vi "set default configuration.vi"(8 "error in":errorcluster, 11 "Shared Memory configuration in":refnum<class "Shared Memory configuration.lvclass">) -> (0 "error out":errorcluster, 3 "Shared Memory configuration out":refnum<class "Shared Memory configuration.lvclass">)   [LabVIEW 2014, in "Shared Memory configuration.lvclass"]
doc: "Initializes configration with default values. Old revisions of the configuration do not update newer fields, so this VI ensures they are set to values that are safe for the runtime execution."
uses:
  Shared Memory configuration.lvclass
  Line.ctl
  <vilib>/NI/Tag Bus Module Framework/channel/TBM channel.lvclass
  editor node/sync/sync item.ctl
  editor node/sync/sync mechanism.ctl
  Shared Memory configuration.lvclass/Shared Memory configuration.ctl
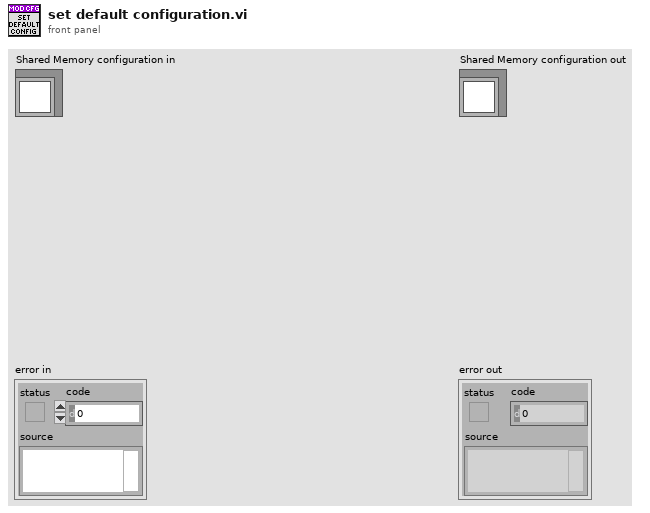
[diagram p1: front panel]
types:
  T1 = typedef "Shared Memory configuration.lvclass/sync item.ctl" = cluster{"mechanism":T2, "name":string}
  T2 = typedef "Shared Memory configuration.lvclass/sync mechanism.ctl" = enum16{"Semaphore"}
  T3 = typedef "Shared Memory configuration.lvclass/Line.ctl" = cluster{"channel":refnum<class "TBM channel.lvclass">}
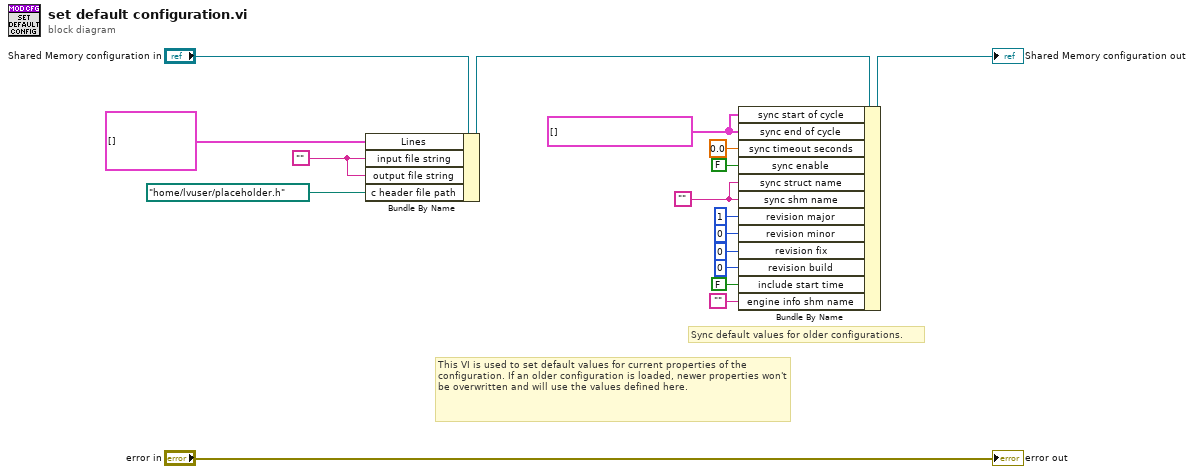
[diagram p0: block diagram]
diagram:
  w12 = T1[] [] ("sync end of cycle")
  w9 = ""
  w14 = ""
  # "This VI is used to set default values for current properties of the configuration. If an older configuration is loaded, newer properties won't be overwritten and will use the values defined here."
  # "Sync default values for older configurations."
  n1 = Bundle By Name(cluster="Shared Memory configuration in", "Lines"=T3[] [], "input file string"=w14, "output file string"=w14, "c header file path"=path "/home/lvuser/placeholder.h" ("c header file directory")) -> (w4:refnum<class "Shared Memory configuration.lvclass">)
  n2 = Bundle By Name(cluster=w4, "sync start of cycle"=w12, "sync end of cycle"=w12, "sync timeout seconds"=0.0, "sync enable"=FALSE, "sync struct name"=w9, "sync shm name"=w9, "revision major"=u8 1, "revision minor"=u8 0, "revision fix"=u8 0, "revision build"=u8 0, "include start time"=FALSE, "engine info shm name"="") -> (→"Shared Memory configuration out":refnum<class "Shared Memory configuration.lvclass">)
  "error out" <- "error in"
